vi "电导率电极校准.vi"() -> ()   [LabVIEW 2016, in "斯坦道多参数.lvlib"]
uses:
  <vilib>/Utility/miscctls.llb/LVPointTypeDef.ctl
  <vilib>/Analysis/NI_AALBase.lvlib
panel:
  out "盐度":dbl caption="盐度测量值" format="%#.2g"
  out "温度":dbl format="%#.2g"
  out "当前信号值":dbl format="%#.2g"
  in  "校准停止":bool
  in  "校准启动":bool
  out "波形图表":sgl(graph) caption="历史曲线"
  out "第二点校准值":dbl
  out "第一点校准值":dbl
  in  "校准模式":enum16{"两点校准", "单点校准"}(ring)=enum."单点校准"
  out "提示":string
  out "最小值":sgl format="%#.2f"
  out "最大值":sgl format="%#.2f"
  out "mean":dbl caption="均值" format="%#.2f"
  out "standard deviation":dbl caption="标准差" format="%#.2f"
  out "变异系数":dbl format="%#.6f"
  out "标液2":dbl
  out "标液1":dbl
  out "当前读取值":dbl caption="当前测试值" format="%#.2g"
  out "电极系数":dbl
  out "偏移值补偿":dbl format="%#.2g"
  out "温度补偿系数":dbl caption="温度系数"
  # "电导率电极设定"
  # "请选择校准模式:"
  # "℃"
  # "uS/cm"
  # "uS/cm"
  # "cm"
  # "-1"
  # "uS/cm"
  # "%"
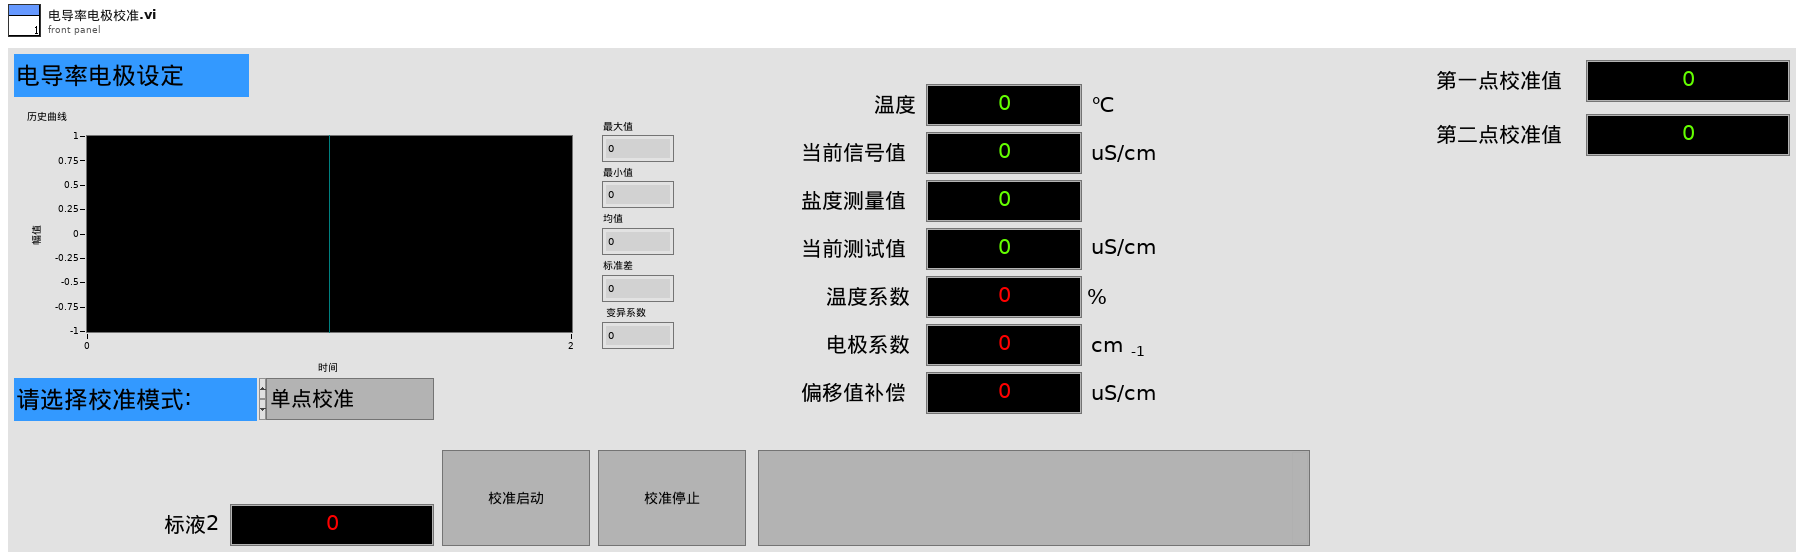
[diagram p1: front panel]
types:
  T1 = typedef "斯坦道多参数.lvlib/校准步骤.ctl" = enum16{"待机", "放置第一点标液", "第一点校准启动", "第一点校准写入", "第一点校准失败", "放置第二点标液", "第二点校准启动", "第二点校准写入", "第二点校准失败", "放置第三点标液", "第三点校准启动", "第三点校准写入", "第三点校准失败", "校准结果写入", "校准结束"}
  T2 = typedef "LVPointTypeDef.ctl" = cluster{"Horizontal":i16, "Vertical":i16}
  T3 = cluster{"电极状态标志":u16, "电极型号标志":u16, "电导率测量值":sgl, "温度测量值":sgl, "电导率信号值":sgl, "温度信号值":sgl, "温度补偿系数":sgl, "电导率偏移修正值":sgl, "温度偏移修正值":sgl, "手动温度补偿值":sgl, "电导率电极零点":sgl, "电导率电极斜率":sgl, "命令滤波设定":u16, "温度模式":enum16{"ATC", "MTC"}, "生产批次":u16, "电极序号":u16, "串口地址":u16, "串口波特率":enum16{"9600", "19200", "115200"}, "串口校验位":enum16{"NONE", "ODD", "EVEN"}, "串口停止位":enum16{"1bit", "2bit"}, "第一点标准值":sgl, "第二点标准值":sgl}
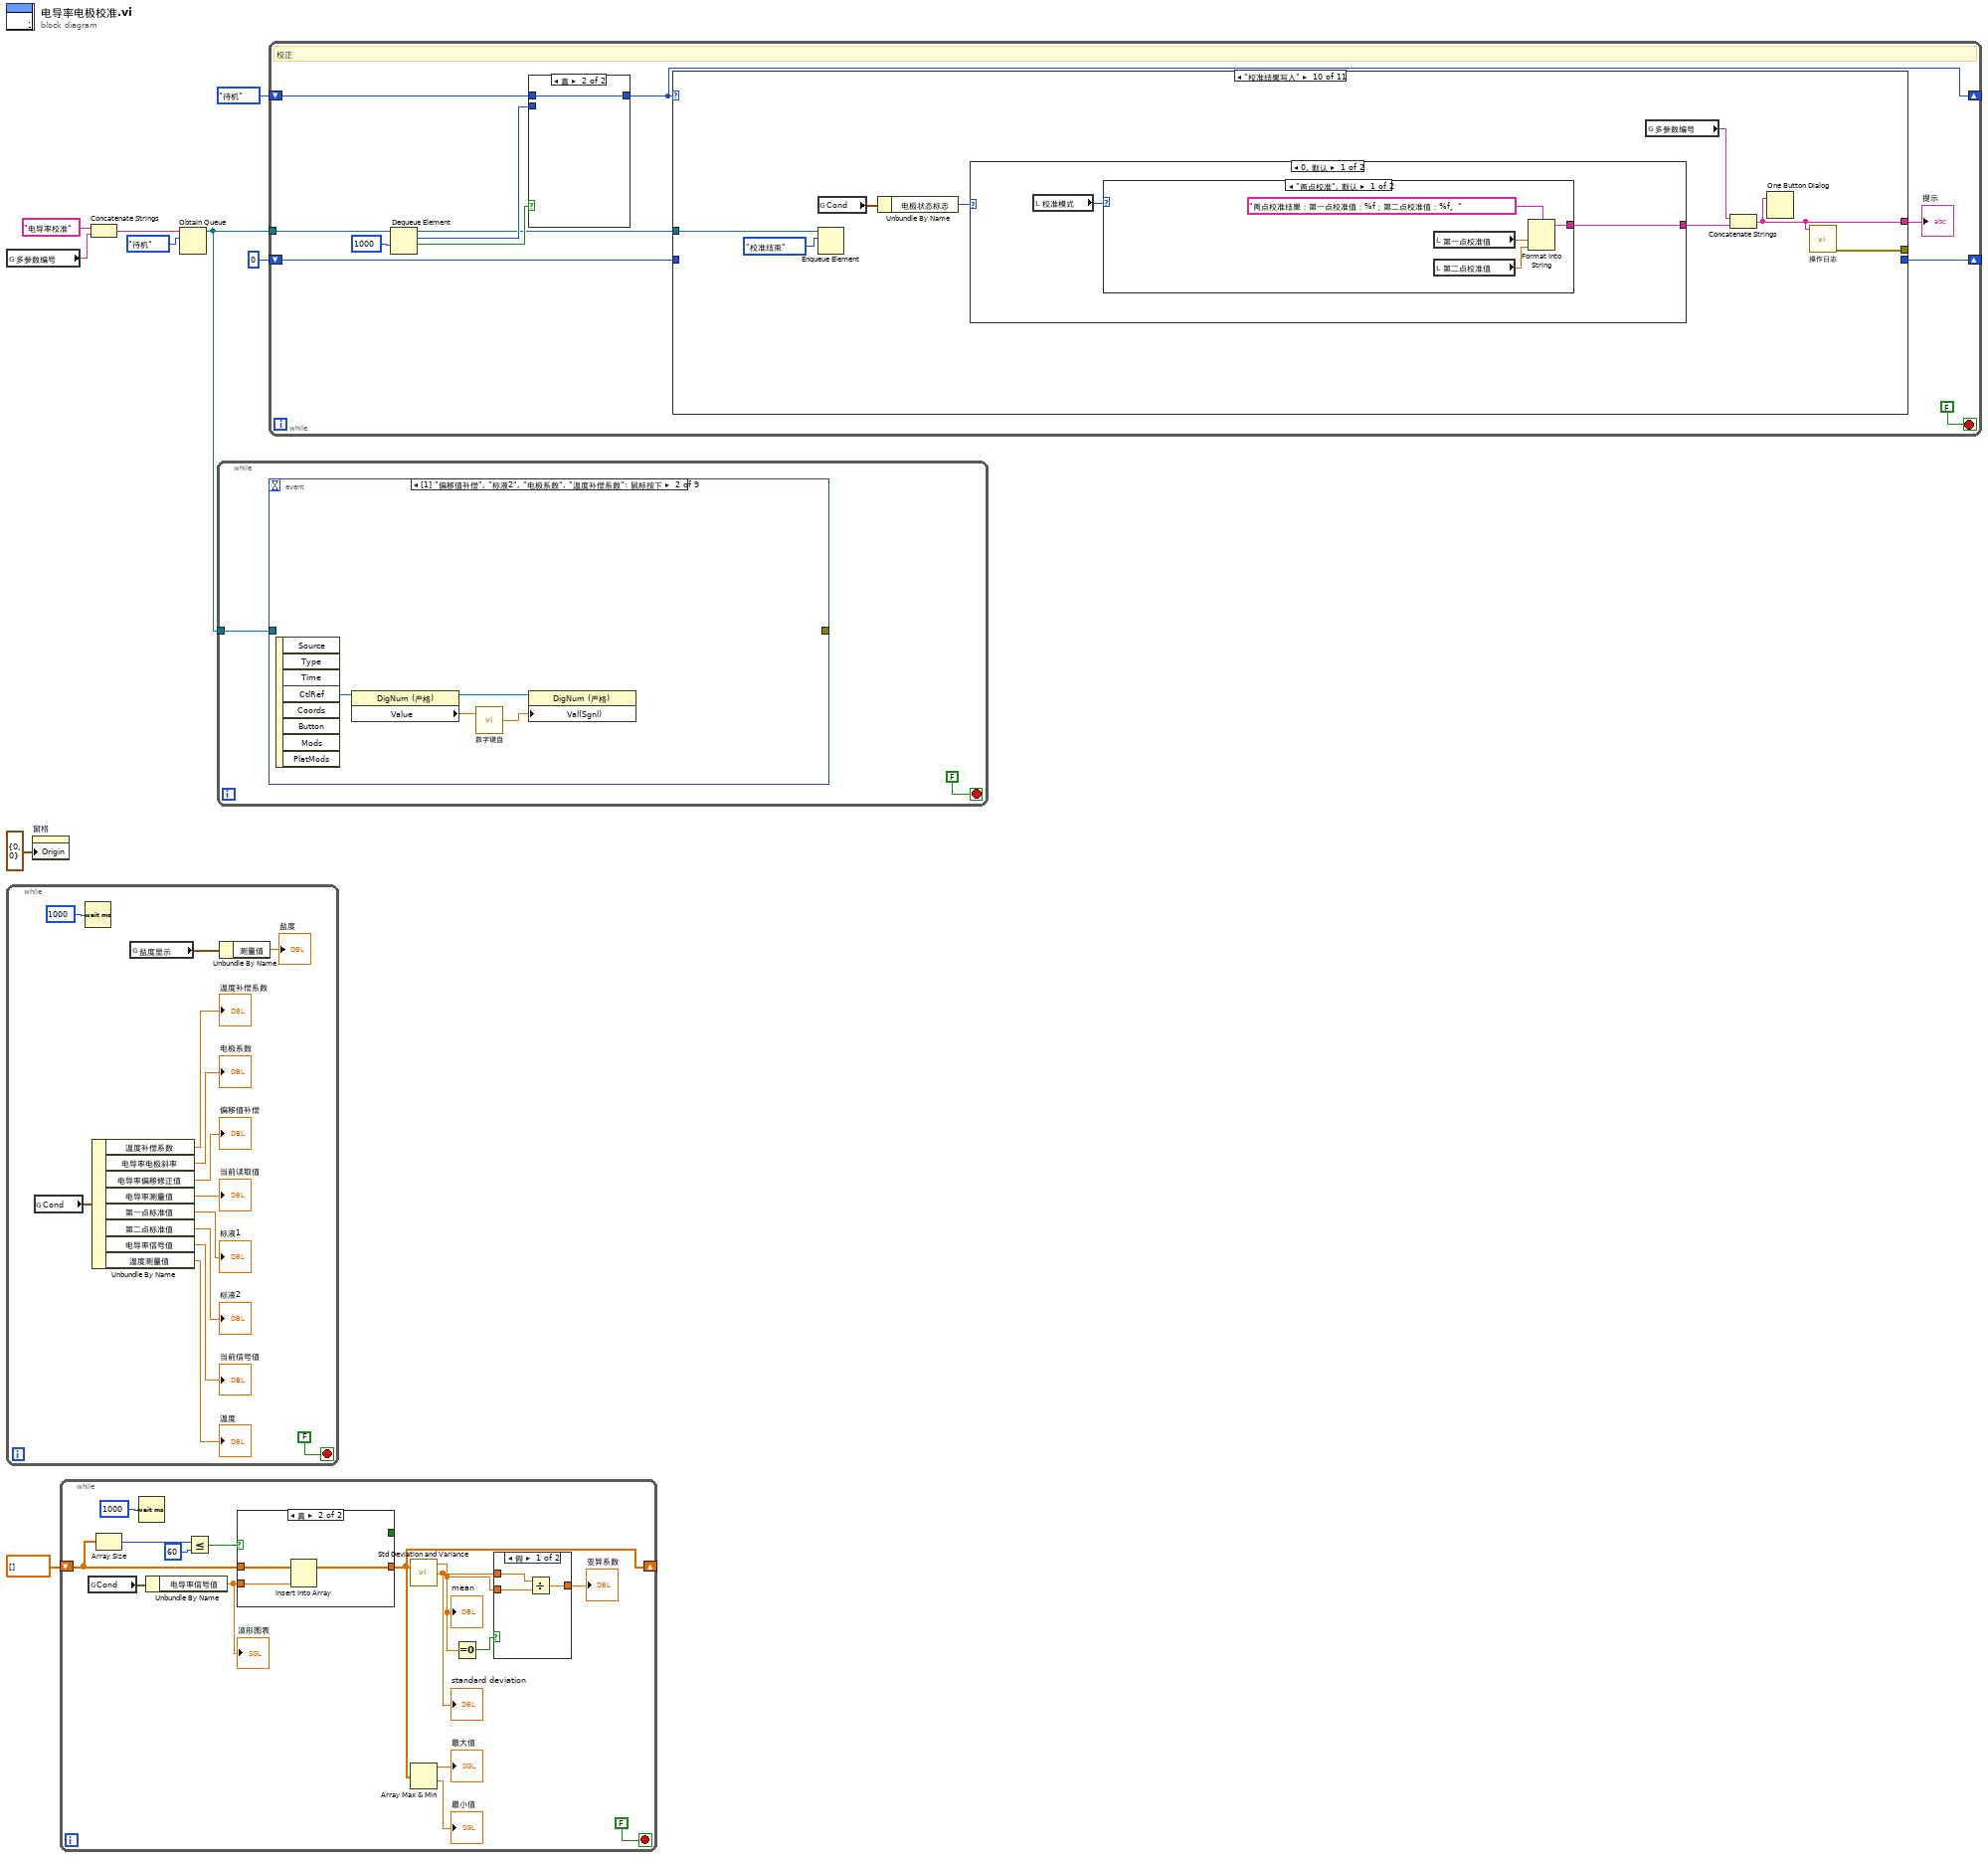
[diagram p0: block diagram]
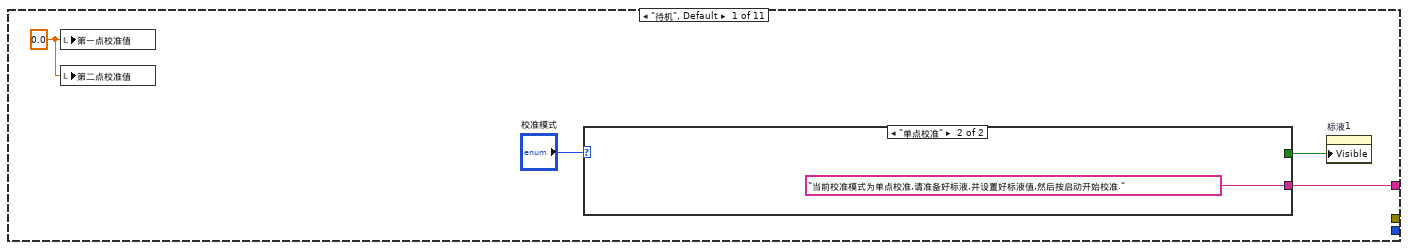
[diagram p3: hidden frame]
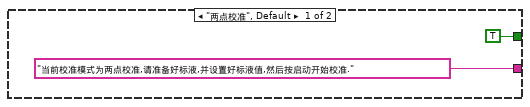
[diagram p4: hidden frame]
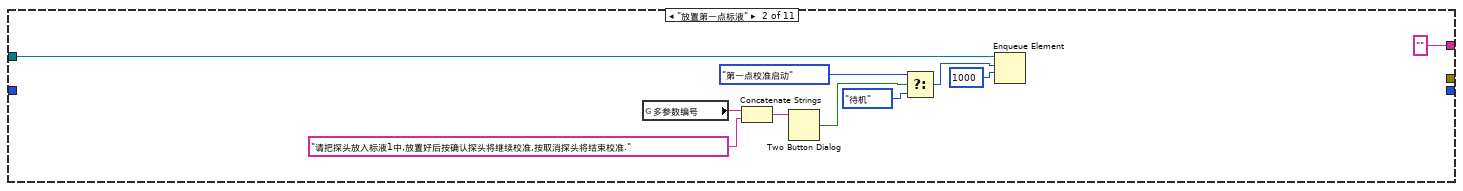
[diagram p5: hidden frame]
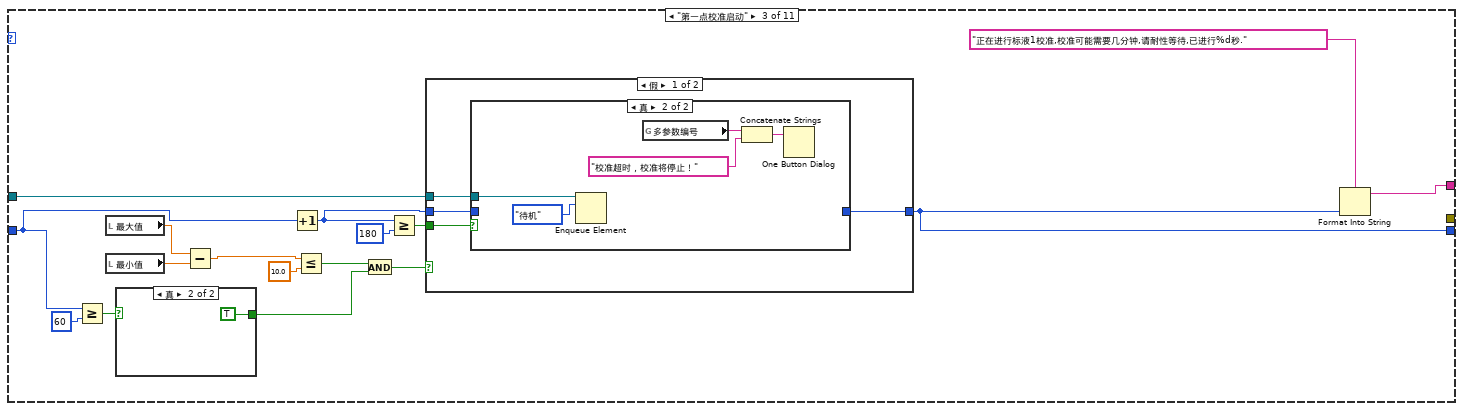
[diagram p6: hidden frame]
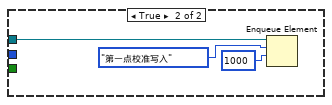
[diagram p8: hidden frame]
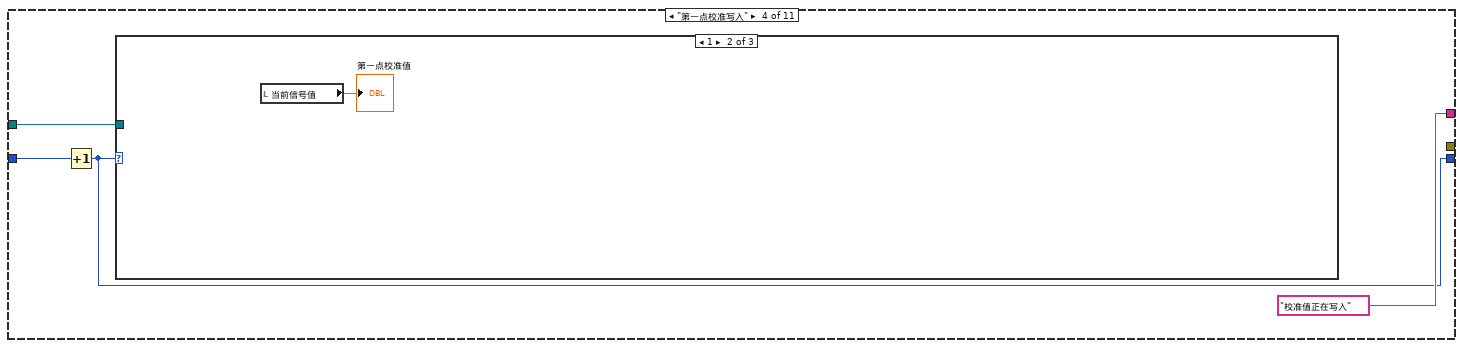
[diagram p10: hidden frame]
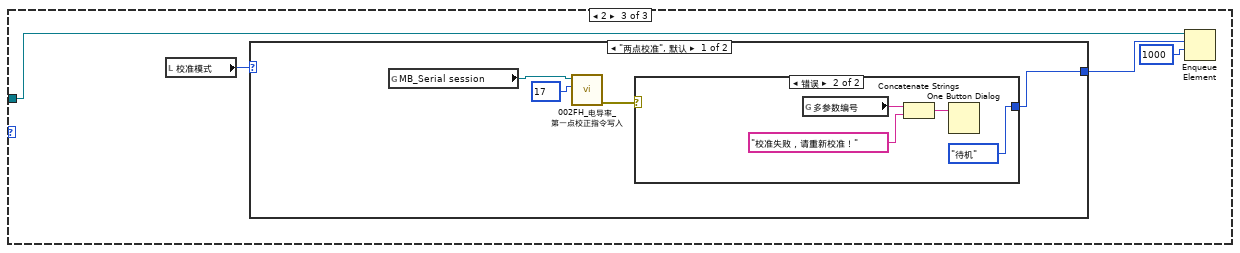
[diagram p12: hidden frame]
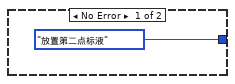
[diagram p13: hidden frame]
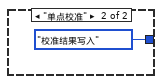
[diagram p14: hidden frame]
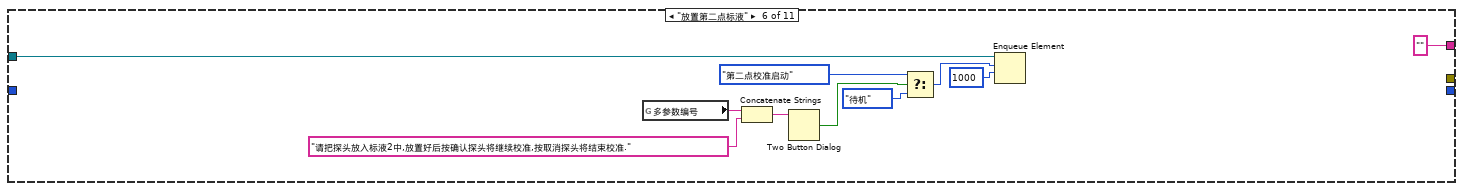
[diagram p16: hidden frame]
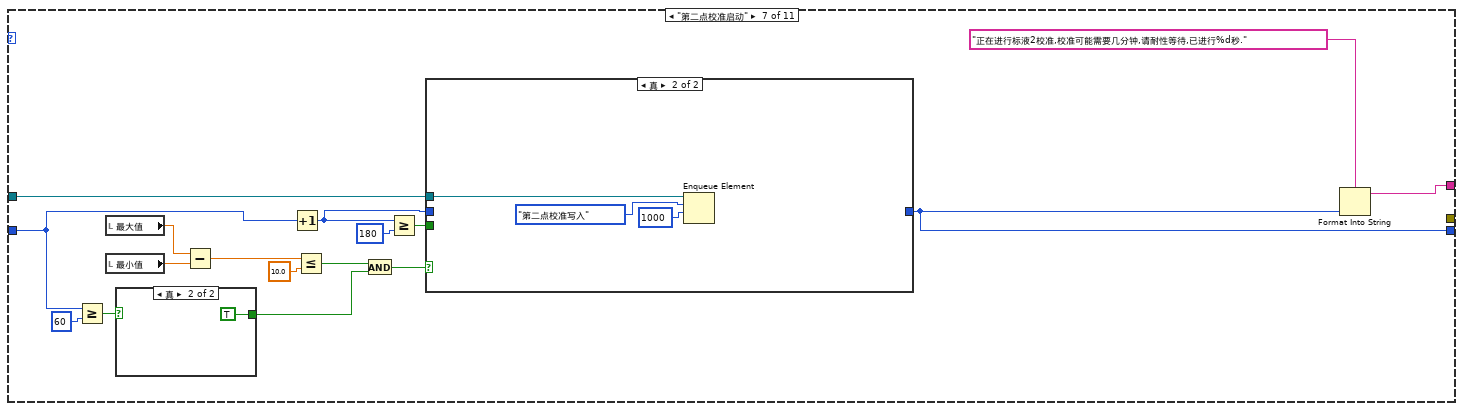
[diagram p17: hidden frame]
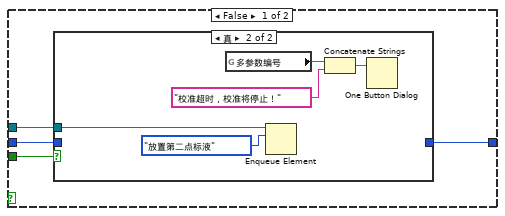
[diagram p18: hidden frame]
diagram:
  n1 = global read "多参数全局变量.vi" "多参数编号"() -> (w1:string)
  n2 = while {
    stop <- FALSE stop-if-true
    n3 = global read "国弘过程全局变量.vi" "Cond"() -> (w20:T3)
    n4 = Wait (ms)(milliseconds to wait=u32 1000 ("等待时间（毫秒）")) -> ()  [unwired: 1 out]
    n5 = Unbundle By Name(w20) -> ("温度补偿系数"=→"温度补偿系数":sgl, "电导率电极斜率"=→"电极系数":sgl, "电导率偏移修正值"=→"偏移值补偿":sgl, "电导率测量值"=→"当前读取值":sgl, "第一点标准值"=→"标液1":sgl, "第二点标准值"=→"标液2":sgl, "电导率信号值"=→"当前信号值":sgl, "温度测量值"=→"温度":sgl)
    n6 = global read "多参数全局变量.vi" "盐度显示"() -> (w11:cluster{"温度测量值":sgl, "测量值":sgl, "温度偏移修正值":sgl})
    n7 = Unbundle By Name(w11) -> ("测量值"=→"盐度":sgl)
  }
  n8 = property on="窗格" class="Pane"("Origin"=T2 {"Horizontal"=0, "Vertical"=0} ("原点")) -> ()  [unwired: 2 in, 2 out]
  n9 = while {
    shift-right: [w26] -> _
    shift-left: sgl[] [] -> [w33]
    stop <- FALSE stop-if-true
    n10 = global read "国弘过程全局变量.vi" "Cond"() -> (w27:T3)
    n11 = Array Size(array=w33) -> (size(s)=w35:i32)
    n12 = Wait (ms)(milliseconds to wait=u32 1000 ("等待时间（毫秒）")) -> ()  [unwired: 1 out]
    n13 = Unbundle By Name(w27) -> ("电导率信号值"=w23:sgl)
    "波形图表" <- w23
    n14 = Less Or Equal?(x=w35, y=60) -> (x <= y?=w34:bool)
    n15 = case shown="真" w34 {
      tunnel: w33 -> [w46 w49]
      tunnel: w23 -> [w44 w48]
      tunnel: [w42 w47] -> w26
      tunnel: [TRUE _] -> _
      frame False {
        n16 = Replace Array Subset(array=w46, new element=w44) -> (w45:sgl[])  [unwired: 1 in]
        n17 = Rotate 1D Array(1:w45, 2:-1 ("n")) -> (0:w42:sgl[])
      }
      frame True {
        n18 = Insert Into Array(array=w49, new element=w48) -> (w47:sgl[])  [unwired: 1 in]
      }
    }
    n19 = call <vilib>:"Std Deviation and Variance.vi"("X"=w26) -> ("mean"=w31:dbl, "standard deviation"=w30:dbl)  [unwired: 1 in, 1 out]
    "mean" <- w31
    "standard deviation" <- w30
    n20 = Array Max & Min(array=w26) -> (max value=→"最大值":sgl, min value=→"最小值":sgl)  [unwired: 2 out]
    n21 = Equal To 0?(x=w31) -> (x = 0?=w32:bool)
    n22 = case shown="假" w32 {
      tunnel: w30 -> [w40 _]
      tunnel: [w39 _] -> w29
      tunnel: w31 -> [w38 _]
      frame False {
        n23 = Divide(x=w40, y=w38) -> (x/y=w39:dbl)
      }
      frame True {
      }
    }
    "变异系数" <- w29
  }
  n24 = Concatenate Strings("电导率校准" ("名称（未命名）"), w1) -> (w2:string)
  n25 = Obtain Queue(name (unnamed)=w2, element data type=校准步骤."待机" ("枚举")) -> (queue out=w3:refnum<queue>)  [unwired: 3 in, 2 out]
  n26 = while {
    tunnel: w3 -> [w50]
    stop <- FALSE stop-if-true
    n27 = event shown="[1] \"偏移值补偿\", \"标液2\", \"电极系数\", \"温度补偿系数\": 鼠标按下" {
      selector: _ -> [_ _ _ _ _ _ _ _ _]
      dyn-events: _ -> [_ _ _ _ _ _ _ _ _]
      timeout: _ -> [_ _ _ _ _ _ _ _ _]
      tunnel: [_ _ w57 w60 w63 w67 w70 _ _] -> _
      tunnel: w50 -> [_ _ _ _ _ _ _ w73 w76]
      event Timeout {
        n28 = event-data() -> ()  [unwired: 1 in, 3 out]
      }
      event "偏移值补偿", "标液2", "电极系数", "温度补偿系数": Mouse Down {
        n29 = event-data() -> ("CtlRef"=w52:refnum<vi>)  [unwired: 1 in, 7 out]
        n30 = property class="DigNum (严格)"(reference=w52) -> (reference out=w53:refnum<vi>, "Value"=w54:dbl)  [unwired: 1 in, 1 out]
        n31 = call "数字键盘.vi"("OldNumber"=w54) -> ("NewNumber"=w55:dbl)  [unwired: 1 in]
        n32 = property class="DigNum (严格)"(reference=w53, "Val(Sgnl)"=w55) -> ()  [unwired: 1 in, 2 out]
      }
      event "温度补偿系数": Value Change {
        n33 = event-data() -> ("NewVal"=w58:dbl)  [unwired: 1 in, 5 out]
        n34 = global read "多参数全局变量.vi" "MB_Serial session"() -> (w56:refnum<class "MB_Master_Serial.lvclass">)
        n35 = call "000AH_电导率_温度补偿系数写入.vi"("数值"=w58, "MB_Serial session in"=w56) -> ("error out"=w57:errorcluster)  [unwired: 8 in, 1 out]
      }
      event "偏移值补偿": Value Change {
        n36 = event-data() -> ("NewVal"=w61:dbl)  [unwired: 1 in, 5 out]
        n37 = global read "多参数全局变量.vi" "MB_Serial session"() -> (w59:refnum<class "MB_Master_Serial.lvclass">)
        n38 = call "000CH_电导率_电导率偏移修正值写入.vi"("数值"=w61, "MB_Serial session in"=w59) -> ("error out"=w60:errorcluster)  [unwired: 8 in, 1 out]
      }
      event "标液1": Value Change {
        n39 = event-data() -> ("NewVal"=w64:dbl)  [unwired: 1 in, 5 out]
        n40 = global read "多参数全局变量.vi" "MB_Serial session"() -> (w62:refnum<class "MB_Master_Serial.lvclass">)
        n41 = call "0030H_电导率_第一点标准值写入.vi"("数值"=w64, "MB_Serial session in"=w62) -> ("error out"=w63:errorcluster)  [unwired: 8 in, 1 out]
      }
      event "标液2": Value Change {
        n42 = event-data() -> ("NewVal"=w66:dbl)  [unwired: 1 in, 5 out]
        n43 = global read "多参数全局变量.vi" "MB_Serial session"() -> (w65:refnum<class "MB_Master_Serial.lvclass">)
        n44 = call "0033H_电导率_第二点标准值写入.vi"("数值"=w66, "MB_Serial session in"=w65) -> ("error out"=w67:errorcluster)  [unwired: 8 in, 1 out]
      }
      event "电极系数": Value Change {
        n45 = event-data() -> ("NewVal"=w69:dbl)  [unwired: 1 in, 5 out]
        n46 = global read "多参数全局变量.vi" "MB_Serial session"() -> (w68:refnum<class "MB_Master_Serial.lvclass">)
        n47 = call "0014H_电导率_电极系数写入.vi"("数值"=w69, "MB_Serial session in"=w68) -> ("error out"=w70:errorcluster)  [unwired: 8 in, 1 out]
      }
      event "校准启动": Value Change {
        n48 = event-data() -> ()  [unwired: 1 in, 6 out]
        n49 = local read "校准模式"() -> (w72:enum16{"两点校准", "单点校准"})
        n50 = case shown="\"两点校准\", 默认" w72 {
          tunnel: [校准步骤."放置第一点标液" ("元素") 校准步骤."放置第二点标液" ("元素")] -> w71
          frame "两点校准", Default {
          }
          frame "单点校准" {
          }
        }
        n51 = Enqueue Element(queue=w73, element=w71) -> ()  [unwired: 2 in, 3 out]
      }
      event "校准停止": Value Change {
        n52 = event-data() -> ()  [unwired: 1 in, 6 out]
        n53 = Flush Queue(queue=w76) -> (queue out=w77:refnum<queue>)  [unwired: 1 in, 2 out]
        n54 = Enqueue Element(queue=w77, element=校准步骤."待机" ("元素"), timeout in ms (-1)=1000 ("超时毫秒(-1)")) -> ()  [unwired: 1 in, 3 out]
      }
    }
  }
  n55 = while "While循环" {
    shift-right: [w81] -> _
    shift-left: 校准步骤."待机" ("枚举") -> [w82]
    shift-right: [w88] -> _
    shift-left: 0 -> [w89]
    tunnel: w3 -> [w86]
    stop <- FALSE stop-if-true
    # "校正"
    n56 = Dequeue Element(queue=w86, timeout in ms (-1)=1000 ("超时毫秒(-1)")) -> (queue out=w80:refnum<queue>, element=w83:T1, timed out?=w84:bool)  [unwired: 1 in, 1 out]
    n57 = case shown="真" w84 {
      tunnel: w83 -> [w91 _]
      tunnel: [w91 w92] -> w81
      tunnel: w82 -> [_ w92]
      frame False {
      }
      frame True {
      }
    }
    n58 = case shown="\"校准结果写入\"" w81 {
      tunnel: [w96 "" ("提示") w125 "校准值正在写入" ("提示") _ "" ("提示") w185 "校准值正在写入" ("提示") _ w218 w235] -> w87
      tunnel: w89 -> [_ _ w119 w143 _ _ w179 w203 _ _ _]
      tunnel: [_ _ w110 w142 _ _ w170 w202 _ _ _] -> w88
      tunnel: w80 -> [_ w108 w113 w141 _ w168 w173 w201 _ w224 _]
      tunnel: [_ _ _ _ _ _ _ _ _ w219 _] -> _
      frame "待机", Default {
        w93 = 0.0 ("第一点校准值")
        n59 = local write "第一点校准值"(w93) -> ()
        n60 = local write "第二点校准值"(w93) -> ()
        n61 = case shown="\"单点校准\"" "校准模式" {
          tunnel: ["当前校准模式为两点校准,请准备好标液,并设置好标液值,然后按启动开始校准." ("提示") "当前校准模式为单点校准,请准备好标液,并设置好标液值,然后按启动开始校准." ("提示")] -> w96
          tunnel: [TRUE ("可见") _] -> w95
          frame "两点校准", Default {
          }
          frame "单点校准" {
          }
        }
        n62 = property on="标液1" class="DigNum (严格)"("Visible"=w95) -> ()  [unwired: 2 in, 2 out]
      }
      frame "放置第一点标液" {
        n63 = global read "多参数全局变量.vi" "多参数编号"() -> (w100:string)
        n64 = Concatenate Strings(w100, "请把探头放入标液1中,放置好后按确认探头将继续校准,按取消探头将结束校准." ("消息")) -> (w101:string)
        n65 = Two Button Dialog(message=w101) -> (T button?=w106:bool)  [unwired: 2 in]
        n66 = Select(t=校准步骤."第一点校准启动" ("元素"), s=w106, f=校准步骤."待机" ("元素")) -> (s? t:f=w103:T1)
        n67 = Enqueue Element(queue=w108, element=w103, timeout in ms (-1)=1000 ("超时毫秒(-1)")) -> ()  [unwired: 1 in, 3 out]
      }
      frame "第一点校准启动" {
        n68 = Greater Or Equal?(x=w119, y=60) -> (x >= y?=w120:bool)
        n69 = local read "最大值"() -> (w116:sgl)
        n70 = local read "最小值"() -> (w117:sgl)
        n71 = case shown="真" w120 {
          tunnel: [_ TRUE] -> w118
          frame False {
          }
          frame True {
          }
        }
        n72 = Subtract(x=w116, y=w117) -> (x-y=w115:sgl)
        n73 = Increment(x=w119) -> (x+1=w111:i32)
        n74 = Less Or Equal?(x=w115, y=10.0) -> (x <= y?=w123:bool)
        n75 = And(x=w123, y=w118) -> (x .and. y?=w114:bool)
        n76 = Greater Or Equal?(x=w111, y=180) -> (x >= y?=w112:bool)
        n77 = case shown="假" w114 {
          tunnel: w113 -> [w129 w139]
          tunnel: w112 -> [w130 _]
          tunnel: w111 -> [w128 _]
          tunnel: [w127 _] -> w110
          frame False {
            n78 = case shown="真" w130 {
              tunnel: w129 -> [_ w136]
              tunnel: w128 -> [w131 _]
              tunnel: [w131 _] -> w127
              frame False {
              }
              frame True {
                n79 = Enqueue Element(queue=w136, element=校准步骤."待机" ("元素")) -> ()  [unwired: 2 in, 3 out]
                n80 = global read "多参数全局变量.vi" "多参数编号"() -> (w132:string)
                n81 = Concatenate Strings(w132, "校准超时，校准将停止！" ("消息")) -> (w133:string)
                n82 = One Button Dialog(message=w133) -> ()  [unwired: 1 in, 1 out]
              }
            }
          }
          frame True {
            n83 = Enqueue Element(queue=w139, element=校准步骤."第一点校准写入" ("元素"), timeout in ms (-1)=1000 ("超时毫秒(-1)")) -> ()  [unwired: 1 in, 3 out]
          }
        }
        n84 = Format Into String(format string="正在进行标液1校准,校准可能需要几分钟,请耐性等待,已进行%d秒." ("格式字符串"), w110) -> (resulting string=w125:string)  [unwired: 2 in, 1 out]
      }
      frame "第一点校准写入" {
        n85 = Increment(x=w143) -> (x+1=w142:i32)
        n86 = case shown="1" w142 {
          tunnel: w141 -> [_ _ w149]
          frame 0, Default {
          }
          frame 1 {
            n87 = local read "当前信号值"() -> (→"第一点校准值":dbl)
          }
          frame 2 {
            n88 = local read "校准模式"() -> (w148:enum16{"两点校准", "单点校准"})
            n89 = case shown="\"两点校准\", 默认" w148 {
              tunnel: [w153 校准步骤."校准结果写入" ("元素")] -> w147
              frame "两点校准", Default {
                n90 = global read "多参数全局变量.vi" "MB_Serial session"() -> (w151:refnum<class "MB_Master_Serial.lvclass">)
                n91 = call "002FH_电导率_第一点校正指令写入.vi"("数值"=u16 17, "MB_Serial session in"=w151) -> ("error out"=w152:errorcluster)  [unwired: 8 in, 1 out]
                n92 = case shown="错误" w152 {
                  tunnel: [校准步骤."放置第二点标液" ("元素") 校准步骤."待机" ("元素")] -> w153
                  frame No Error {
                  }
                  frame Error {
                    n93 = global read "多参数全局变量.vi" "多参数编号"() -> (w155:string)
                    n94 = Concatenate Strings(w155, "校准失败，请重新校准！" ("消息")) -> (w156:string)
                    n95 = One Button Dialog(message=w156) -> ()  [unwired: 1 in, 1 out]
                  }
                }
              }
              frame "单点校准" {
              }
            }
            n96 = Enqueue Element(queue=w149, element=w147, timeout in ms (-1)=1000 ("超时毫秒(-1)")) -> ()  [unwired: 1 in, 3 out]
          }
        }
      }
      frame "第一点校准失败" {
      }
      frame "放置第二点标液" {
        n97 = global read "多参数全局变量.vi" "多参数编号"() -> (w160:string)
        n98 = Concatenate Strings(w160, "请把探头放入标液2中,放置好后按确认探头将继续校准,按取消探头将结束校准." ("消息")) -> (w161:string)
        n99 = Two Button Dialog(message=w161) -> (T button?=w166:bool)  [unwired: 2 in]
        n100 = Select(t=校准步骤."第二点校准启动" ("元素"), s=w166, f=校准步骤."待机" ("元素")) -> (s? t:f=w163:T1)
        n101 = Enqueue Element(queue=w168, element=w163, timeout in ms (-1)=1000 ("超时毫秒(-1)")) -> ()  [unwired: 1 in, 3 out]
      }
      frame "第二点校准启动" {
        n102 = Greater Or Equal?(x=w179, y=60) -> (x >= y?=w180:bool)
        n103 = local read "最大值"() -> (w176:sgl)
        n104 = local read "最小值"() -> (w177:sgl)
        n105 = case shown="真" w180 {
          tunnel: [_ TRUE] -> w178
          frame False {
          }
          frame True {
          }
        }
        n106 = Subtract(x=w176, y=w177) -> (x-y=w175:sgl)
        n107 = Increment(x=w179) -> (x+1=w171:i32)
        n108 = Less Or Equal?(x=w175, y=10.0) -> (x <= y?=w183:bool)
        n109 = And(x=w183, y=w178) -> (x .and. y?=w174:bool)
        n110 = Greater Or Equal?(x=w171, y=180) -> (x >= y?=w172:bool)
        n111 = case shown="真" w174 {
          tunnel: w173 -> [w189 w199]
          tunnel: w172 -> [w190 _]
          tunnel: w171 -> [w188 _]
          tunnel: [w187 _] -> w170
          frame False {
            n112 = case shown="真" w190 {
              tunnel: w189 -> [_ w196]
              tunnel: w188 -> [w191 _]
              tunnel: [w191 _] -> w187
              frame False {
              }
              frame True {
                n113 = global read "多参数全局变量.vi" "多参数编号"() -> (w192:string)
                n114 = Enqueue Element(queue=w196, element=校准步骤."放置第二点标液" ("元素")) -> ()  [unwired: 2 in, 3 out]
                n115 = Concatenate Strings(w192, "校准超时，校准将停止！" ("消息")) -> (w193:string)
                n116 = One Button Dialog(message=w193) -> ()  [unwired: 1 in, 1 out]
              }
            }
          }
          frame True {
            n117 = Enqueue Element(queue=w199, element=校准步骤."第二点校准写入" ("元素"), timeout in ms (-1)=1000 ("超时毫秒(-1)")) -> ()  [unwired: 1 in, 3 out]
          }
        }
        n118 = Format Into String(format string="正在进行标液2校准,校准可能需要几分钟,请耐性等待,已进行%d秒." ("格式字符串"), w170) -> (resulting string=w185:string)  [unwired: 2 in, 1 out]
      }
      frame "第二点校准写入" {
        n119 = Increment(x=w203) -> (x+1=w202:i32)
        n120 = case shown="1" w202 {
          tunnel: w201 -> [_ _ w211]
          frame 0, Default {
          }
          frame 1 {
            n121 = local read "当前信号值"() -> (→"第二点校准值":dbl)
          }
          frame 2 {
            n122 = global read "多参数全局变量.vi" "MB_Serial session"() -> (w208:refnum<class "MB_Master_Serial.lvclass">)
            n123 = call "0032H_电导率_第二点校正指令写入.vi"("数值"=u16 33, "MB_Serial session in"=w208) -> ("error out"=w206:errorcluster)  [unwired: 8 in, 1 out]
            n124 = case shown="错误" w206 {
              tunnel: [校准步骤."校准结果写入" ("元素") 校准步骤."放置第二点标液" ("元素")] -> w209
              frame No Error {
              }
              frame Error {
                n125 = global read "多参数全局变量.vi" "多参数编号"() -> (w213:string)
                n126 = Concatenate Strings(w213, "校准失败，请重新校准！" ("消息")) -> (w214:string)
                n127 = One Button Dialog(message=w214) -> ()  [unwired: 1 in, 1 out]
              }
            }
            n128 = Enqueue Element(queue=w211, element=w209, timeout in ms (-1)=1000 ("超时毫秒(-1)")) -> ()  [unwired: 1 in, 3 out]
          }
        }
      }
      frame "第二点校准失败" {
      }
      frame "校准结果写入" {
        n129 = global read "国弘过程全局变量.vi" "Cond"() -> (w222:T3)
        n130 = Enqueue Element(queue=w224, element=校准步骤."校准结束" ("元素")) -> ()  [unwired: 2 in, 3 out]
        n131 = Unbundle By Name(w222) -> ("电极状态标志"=w221:u16)
        n132 = case shown="0, 默认" w221 {
          tunnel: [w226 "校准失败"] -> w220
          frame 0, Default {
            n133 = local read "校准模式"() -> (w225:enum16{"两点校准", "单点校准"})
            n134 = case shown="\"两点校准\", 默认" w225 {
              tunnel: [w227 w231] -> w226
              frame "两点校准", Default {
                n135 = local read "第一点校准值"() -> (w229:dbl)
                n136 = local read "第二点校准值"() -> (w230:dbl)
                n137 = Format Into String(format string="两点校准结果：第一点校准值：%f；第二点校准值：%f。" ("提示"), w229, w230) -> (resulting string=w227:string)  [unwired: 2 in, 1 out]
              }
              frame "单点校准" {
                n138 = local read "第二点校准值"() -> (w233:dbl)
                n139 = Format Into String(format string="校准结果：校准值：%f" ("提示"), w233) -> (resulting string=w231:string)  [unwired: 2 in, 1 out]
              }
            }
          }
          frame 3, 4 {
          }
        }
        n140 = global read "多参数全局变量.vi" "多参数编号"() -> (w217:string)
        n141 = Concatenate Strings(w217, w220) -> (w218:string)
        n142 = One Button Dialog(message=w218) -> ()  [unwired: 1 in, 1 out]
        n143 = call "操作日志.vi"("日志信息"=w218) -> ("error out"=w219:errorcluster)  [unwired: 10 in]
      }
      frame "校准结束" {
        n144 = local read "提示"() -> (w235:string)
      }
    }
    "提示" <- w87
  }
